vi "Drive Motor Controler.vi"   [LabVIEW 2009]
uses:
  Motor Encoder Global.vi
  Drive Control Global DO NOT MODIFY!.vi
  <vilib>/Platform/TimedLoop/XDataNode/XDataNode.xnode
  <vilib>/Platform/TimedLoop/XDataNode/loadlvalarms.vi
  <vilib>/Platform/TimedLoop/XDataNode/timing_clust.ctl
  <vilib>/Platform/TimedLoop/XDataNode/nitl_modes.ctl
  <vilib>/Platform/TimedLoop/XDataNode/wakeup.ctl
  Motor Output Global.vi
  <vilib>/Platform/TimedLoop/XDataNode/XDNodeRunTimeDep.lvlib
types:
  T1 = typedef "XDNodeRunTimeDep.lvlib/timing_clust.ctl" = cluster{"Expected End [f-1]":u64, "Actual End [f-1]":u64, "Finished Late? [f-1]":bool, "Expected End [i-1]":u64, "Actual End [i-1]":u64, "Finished Late? [i-1]":bool, "Expected Start [i]":u64, "Actual Start [i]":u64, "Expected Start [f]":u64, "Actual Start [f]":u64, "Source Name":string, "Structure Name":string, "Period":i64, "Deadline":i64, "Offset":i64, "Start":i64, "Priority":i32, "Timeout":i32, "Mode":T2, "Wakeup Reason":T3, "Error":errorcluster, "Source Type":string, "Secondary Source Type":string, "Global End Time":u64, "Global Start Time":u64, "Frame Duration":u64, "Iteration Duration":u64, "Assigned CPU":i32, "I/O Scan Engine Mode":u32}
  T2 = typedef "XDNodeRunTimeDep.lvlib/nitl_modes.ctl" = enum32{"No Change", "Process missed periods, maintain original phase", "Discard missed periods, maintain original phase", "Process missed periods, ignore original phase", "Discard missed periods, ignore original phase"}
  T3 = typedef "XDNodeRunTimeDep.lvlib/wakeup.ctl" = enum32{"Normal", "Aborted", "Asynchronous wakeup", "Timing source error", "Timed loop error", "Timeout"}
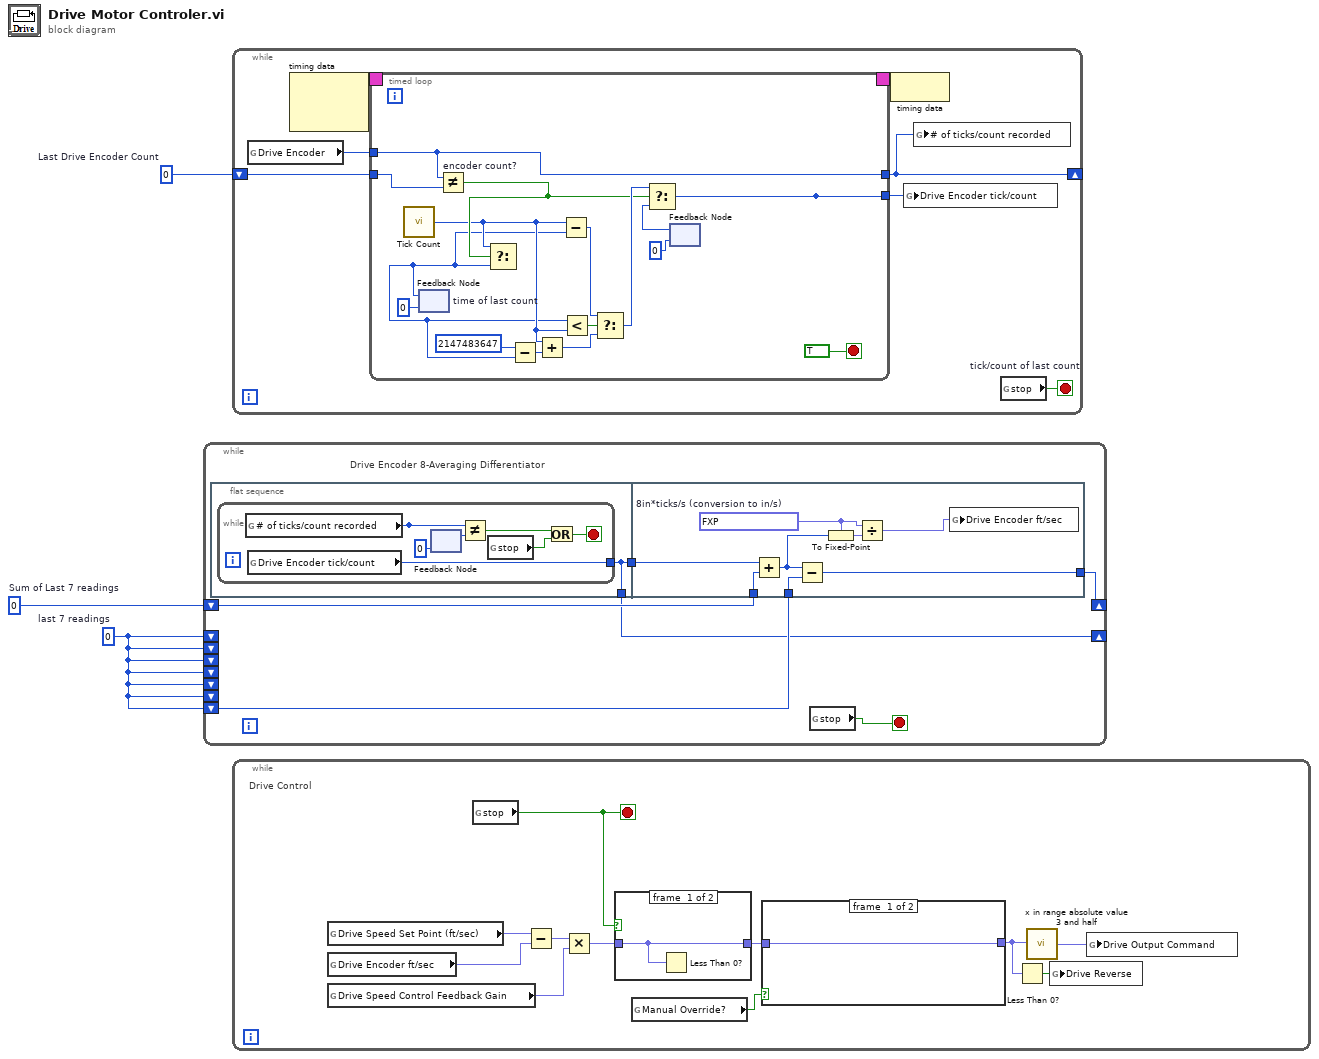
[diagram p0: block diagram]
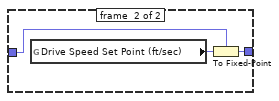
[diagram p2: hidden frame]
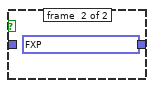
[diagram p3: hidden frame]
diagram:
  w1 = 0  # Last Drive Encoder Count
  w2 = 0  # last 7 readings
  w3 = 0  # Sum of Last 7 readings
  n1 = while {
    shift-right: [w9] -> _
    shift-left: w3 -> [w6]
    shift-right: [w4] -> _
    shift-left: w2 -> [_]
    shift-left: w2 -> [_]
    shift-left: w2 -> [_]
    shift-left: w2 -> [_]
    shift-left: w2 -> [_]
    shift-left: w2 -> [_]
    shift-left: w2 -> [w8]
    stop <- w5 stop-if-true
    # "Drive Encoder 8-Averaging Differentiator"
    n2 = flat-sequence {
      tunnel: [w10] -> w7
      tunnel: [w10] -> w4
      tunnel: [w23] -> w9
      tunnel: w8 -> [w22]
      tunnel: w7 -> [w21]
      tunnel: w6 -> [w20]
      frame #0 {
        n3 = while {
          tunnel: [w15] -> w10
          stop <- w11 stop-if-true
          n4 = global read "Drive Control Global DO NOT MODIFY!.vi" "# of ticks/count recorded"() -> (w14:i32)
          n5 = global read "Drive Control Global DO NOT MODIFY!.vi" "Drive Encoder tick/count"() -> (w15:u32)
          n6 = feedback #1(0 ("Drive Encoder tick/count")) -> (w17:i32)
          n7 = Not Equal?(x=w14, y=w17) -> (x != y?=w12:bool)
          n8 = global read "Motor Encoder Global.vi" "stop"() -> (w13:bool)
          n9 = Or(x=w12, y=w13) -> (x .or. y?=w11:bool)
        }
      }
      frame #1 {
        w18 = fxp<+,31,21> 1387360.33984375  # 8in*ticks/s (conversion to in/s)
        n10 = Add(x=w21, y=w20) -> (x+y=w24:u32)
        n11 = Subtract(x=w24, y=w22) -> (x-y=w23:u32)
        n12 = To Fixed-Point(fixed-point type=w18, number=w24) -> (fixed-point=w25:fxp<+,31,21>)
        n13 = Divide(x=w18, y=w25) -> (x/y=w19:fxp<+/-,18,8>)
        n14 = global write "Drive Control Global DO NOT MODIFY!.vi" "Drive Encoder ft/sec"(w19) -> ()
      }
    }
    n15 = global read "Motor Encoder Global.vi" "stop"() -> (w5:bool)
  }
  n16 = while {
    shift-right: [w27] -> _
    shift-left: w1 -> [w28]
    stop <- w29 stop-if-true
    n17 = global read "Motor Encoder Global.vi" "Drive Encoder"() -> (w26:i32)
    n18 = node-c288() -> (w32:T1)  [unwired: 2 in]
    n19 = timed-loop {
      timing: w32 -> [_]
      timing-out: [_] -> w31
      tunnel: [w34] -> w30
      tunnel: w26 -> [w33]
      tunnel: w28 -> [w49]
      tunnel: [w33] -> w27
      stop <- TRUE stop-if-true
      n20 = call "Tick Count"() -> ("Tick Count(Ticks)"=w39:u32)
      n21 = feedback #2 "time of last count"(u32 0 ("Tick Count(Ticks)")) -> (w36:u32)
      n22 = Not Equal? "encoder count?"(x=w33, y=w49) -> (x != y?=w40:bool)
      n23 = Select(t=w39, s=w40, f=w36) -> (s? t:f=w37:u32)
      n24 = Subtract(x=u32 2147483647, y=w36) -> (x-y=w47:u32)
      n25 = Add(x=w39, y=w47) -> (x+y=w45:u32)
      n26 = Subtract(x=w39, y=w36) -> (x-y=w46:u32)
      n27 = Less?(x=w36, y=w39) -> (x < y?=w41:bool)
      n28 = Select(t=w46, s=w41, f=w45) -> (s? t:f=w44:u32)
      n29 = feedback #3 "tick/count of last count"(u32 0) -> (w43:u32)
      n30 = Select(t=w44, s=w40, f=w43) -> (s? t:f=w34:u32)
    }
    n31 = node-c288(w31) -> ()
    n32 = global write "Drive Control Global DO NOT MODIFY!.vi" "Drive Encoder tick/count"(w30) -> ()
    n33 = global write "Drive Control Global DO NOT MODIFY!.vi" "# of ticks/count recorded"(w27) -> ()
    n34 = global read "Motor Encoder Global.vi" "stop"() -> (w29:bool)
  }
  n35 = while {
    stop <- w59 stop-if-true
    # "Drive Control"
    n36 = global read "Motor Encoder Global.vi" "Drive Speed Set Point (ft/sec)"() -> (w61:fxp<+/-,14,4>)
    n37 = global read "Drive Control Global DO NOT MODIFY!.vi" "Drive Encoder ft/sec"() -> (w62:fxp<+/-,18,8>)
    n38 = global read "Motor Encoder Global.vi" "Drive Speed Control Feedback Gain"() -> (w60:fxp<+/-,20,5>)
    n39 = global read "Motor Encoder Global.vi" "stop"() -> (w59:bool)
    n40 = Subtract(x=w61, y=w62) -> (x-y=w64:fxp<+/-,20,5>)
    n41 = Multiply(x=w64, y=w60) -> (x*y=w63:fxp<+/-,20,5>)
    n42 = case shown="False" w59 {
      tunnel: w63 -> [w69 _]
      tunnel: [w69 fxp<+/-,20,5> 0.0] -> w58
      frame #0 {
        n43 = Less Than 0?(x=w69) -> ()  [unwired: 1 out]
      }
      frame #1 {
      }
    }
    n44 = global read "Motor Output Global.vi" "Manual Override?"() -> (w56:bool)
    n45 = case shown="False" w56 {
      tunnel: [w65 w67] -> w55
      tunnel: w58 -> [w65 w66]
      frame #0 {
      }
      frame #1 {
        n46 = global read "Motor Encoder Global.vi" "Drive Speed Set Point (ft/sec)"() -> (w68:fxp<+/-,14,4>)
        n47 = To Fixed-Point(fixed-point type=w66, number=w68) -> (fixed-point=w67:fxp<+/-,20,5>)
      }
    }
    n48 = Less Than 0?(x=w55) -> (x < 0?=w57:bool)
    n49 = call "x in range absolute value 3 and half.vi"("Numeric"=w55) -> ("y"=w54:fxp<+/-,20,5>)
    n50 = global write "Motor Output Global.vi" "Drive Reverse"(w57) -> ()
    n51 = global write "Motor Output Global.vi" "Drive Output Command"(w54) -> ()
  }
